vi "BusB Mode Word Decode and Update.vi"(0 "BusB":T1, 5 "input bytes":u8[](array[numeric]) format="%x") -> (6 "BusB out":T1, 8 "Sentence Selection":u32, 10 "Boolean array":bool[](array[boolean]))   [LabVIEW 2016, in "Impedance Data Acquisition and Decoding.lvlib"]
uses:
  Impedance Data Acquisition and Decoding.lvlib
  BusB Typedef.ctl
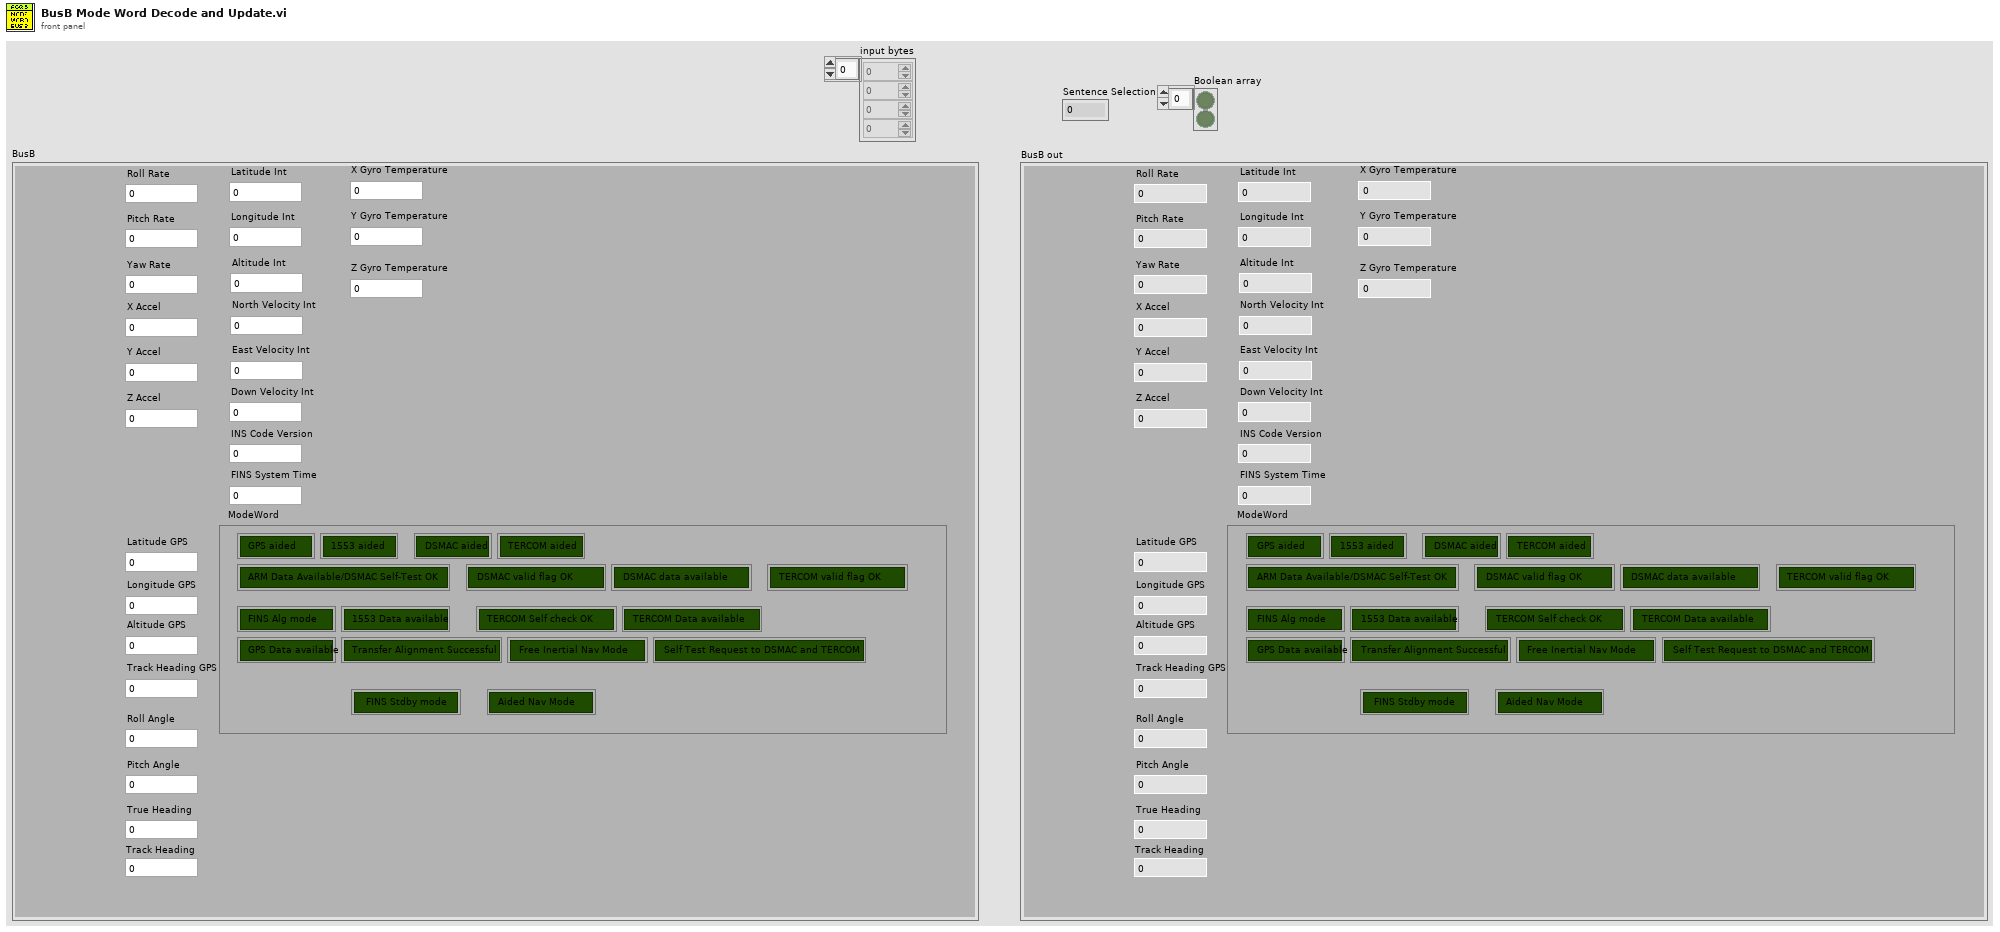
[diagram p1: front panel]
types:
  T1 = typedef "Impedance Data Acquisition and Decoding.lvlib/BusB Typedef.ctl" = cluster{"Pitch Rate":dbl, "Roll Rate":dbl, "Roll Angle":dbl, "Yaw Rate":dbl, "True Heading":dbl, "Pitch Angle":dbl, "Y Accel":dbl, "X Accel":dbl, "Z Accel":dbl, "X Gyro Temperature":dbl, "Longitude GPS":dbl, "Latitude GPS":dbl, "Altitude GPS":dbl, "Track Heading GPS":dbl, "Longitude Int":dbl, "Latitude Int":dbl, "Altitude Int":dbl, "FINS System Time":dbl, "East Velocity Int":dbl, "North Velocity Int":dbl, "INS Code Version":dbl, "ModeWord":cluster{"FINS Alg mode":bool, "GPS Data available":bool, "1553 Data available":bool, "Transfer Alignment Successful":bool, "TERCOM Self check OK":bool, "Free Inertial Nav Mode":bool, "TERCOM Data available":bool, "Self Test Request to DSMAC and TERCOM":bool, "ARM Data Available/DSMAC Self-Test OK":bool, "DSMAC valid flag OK":bool, "DSMAC data available":bool, "TERCOM valid flag OK":bool, "GPS aided":bool, "1553 aided":bool, "DSMAC aided":bool, "TERCOM aided":bool, "Aided Nav Mode":bool, " FINS Stdby mode":bool}, "Down Velocity Int":dbl, "Track Heading":dbl, "Y Gyro Temperature":dbl, "Z Gyro Temperature":dbl}
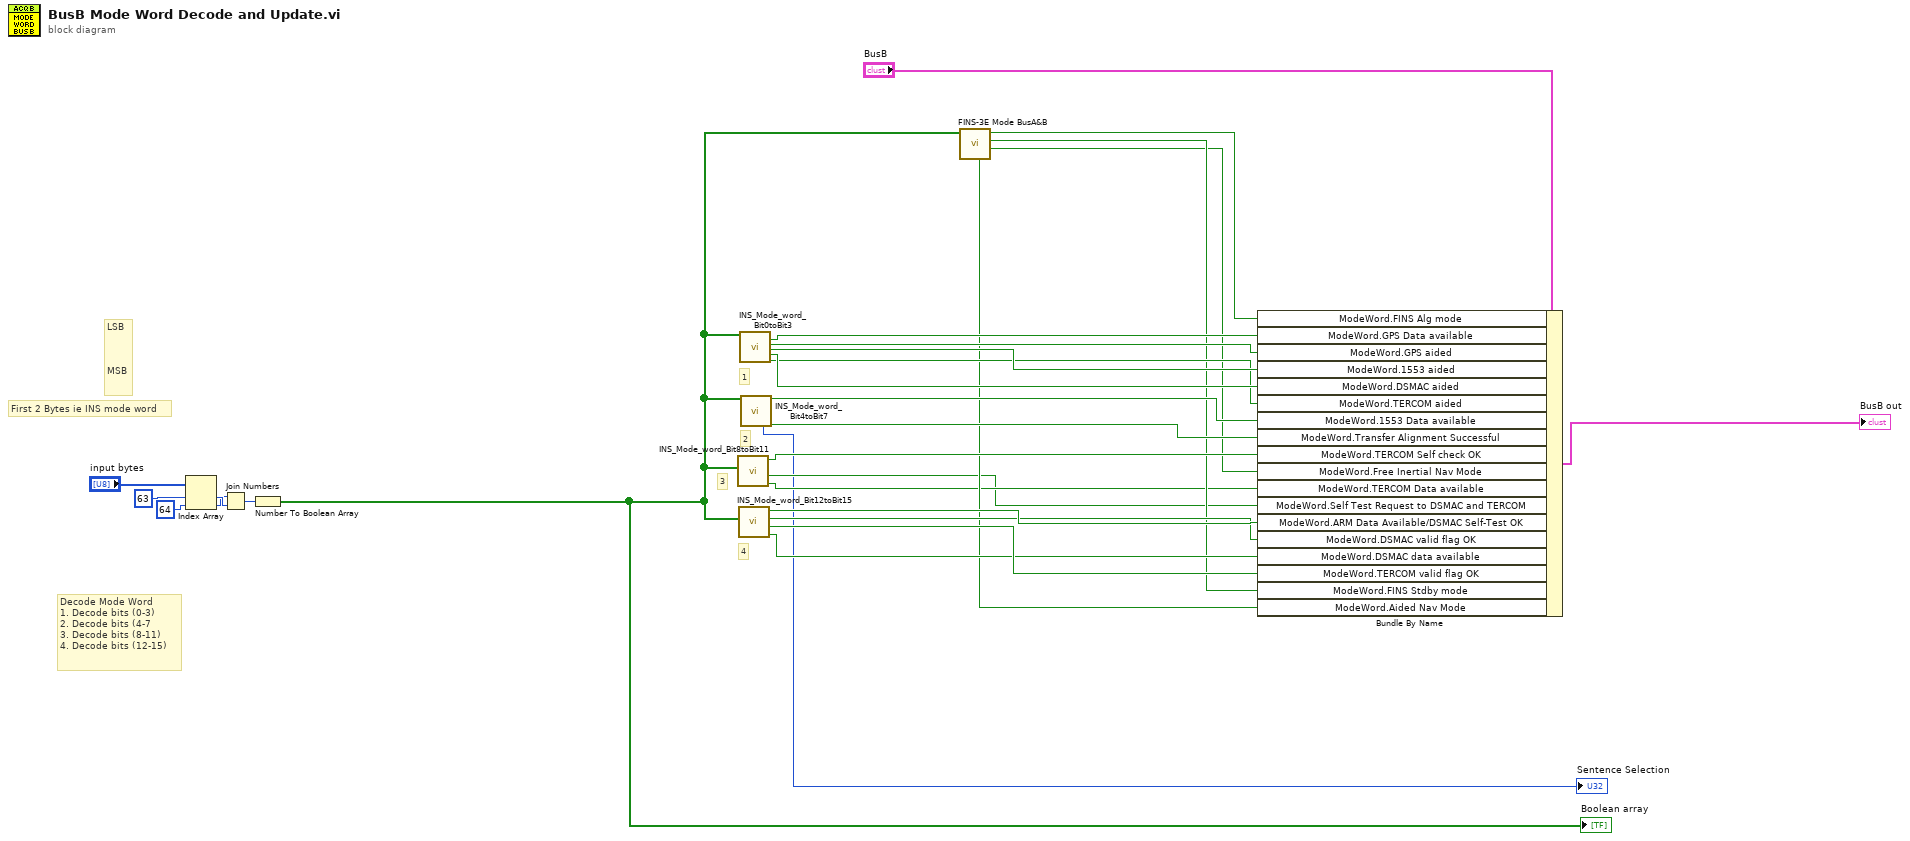
[diagram p0: block diagram]
diagram:
  # "4"
  # "3"
  # "2"
  # "1"
  # "Decode Mode Word\n1. Decode bits (0-3)\n2. Decode bits (4-7\n3. Decode bits (8-11)\n4. Decode bits (12-15)"
  # "LSB\n\n\n\nMSB"
  # "First 2 Bytes ie INS mode word"
  n1 = Index Array(array="input bytes", index #1=63 ("index"), index #2=64 ("index")) -> (element #1=w25:u8, element #2=w24:u8)
  n2 = Join Numbers(hi=w24, lo=w25) -> ((hi.lo)=w23:u16)
  n3 = Number To Boolean Array(number=w23) -> (Boolean array=w2:bool[])
  "Boolean array" <- w2
  n4 = call "INS_Mode_word_Bit8toBit11.vi"("array"=w2) -> ("TERCOM Data Available?"=w6:bool, "Self Test Request to DSMAC and TERCOM"=w5:bool, "TERCOM Self Check OK?"=w15:bool)  [unwired: 7 in, 1 out]
  n5 = call "INS_Mode_word_Bit12toBit15.vi"("array"=w2) -> ("DSMAC Data Available?"=w11:bool, "TERCOm Valid Flag OK?"=w12:bool, "DSMAC Valid Flag OK?"=w13:bool, "Either DSMAC or TERCOM self Check OK Data Out to both DSMAC & TERCOM"=w14:bool)  [unwired: 7 in]
  n6 = call "INS_Mode_word_Bit0toBit3.vi"("array"=w2) -> ("GPS Data Available?"=w22:bool, "GPS Aided ?"=w21:bool, "1553 Aided ?"=w20:bool, "DSMAC Aided ?"=w19:bool, "TERCOM Aided ?"=w18:bool)  [unwired: 12 in, 2 out]
  n7 = call "INS_Mode_word_Bit4toBit7.vi"("array"=w2) -> ("Sentence Selection"=→"Sentence Selection":u32, "1553 Data Available?"=w17:bool, "Transfer Align Succesful?"=w16:bool)  [unwired: 12 in, 4 out]
  n8 = call "FINS-3E Mode BusA&B.vi"("Boolean array"=w2) -> ("Nav, Free Inertial"=w8:bool, "STBY"=w9:bool, "ALG"=w10:bool, "Nav Aided"=w7:bool)  [unwired: 7 in]
  n9 = Bundle By Name(cluster="BusB", "ModeWord.FINS Alg mode"=w10, "ModeWord.GPS Data available"=w22, "ModeWord.GPS aided"=w21, "ModeWord.1553 aided"=w20, "ModeWord.DSMAC aided"=w19, "ModeWord.TERCOM aided"=w18, "ModeWord.1553 Data available"=w17, "ModeWord.Transfer Alignment Successful"=w16, "ModeWord.TERCOM Self check OK"=w15, "ModeWord.Free Inertial Nav Mode"=w8, "ModeWord.TERCOM Data available"=w6, "ModeWord.Self Test Request to DSMAC and TERCOM"=w5, "ModeWord.ARM Data Available/DSMAC Self-Test OK"=w14, "ModeWord.DSMAC valid flag OK"=w13, "ModeWord.DSMAC data available"=w11, "ModeWord.TERCOM valid flag OK"=w12, "ModeWord.FINS Stdby mode"=w9, "ModeWord.Aided Nav Mode"=w7) -> (→"BusB out":T1)
